vi "NEW_PRN Generation_Station1.vi"(8 "error in (no error)":errorcluster, 11 "ClusterIN":T2) -> (0 "error out":errorcluster, 2 "ClusterOUT":T2)   [LabVIEW 2017]
uses:
  <vilib>/addons/database/Connection.llb/Conn ObjectReference.ctl
  <vilib>/addons/database/NI_Database_API.lvlib
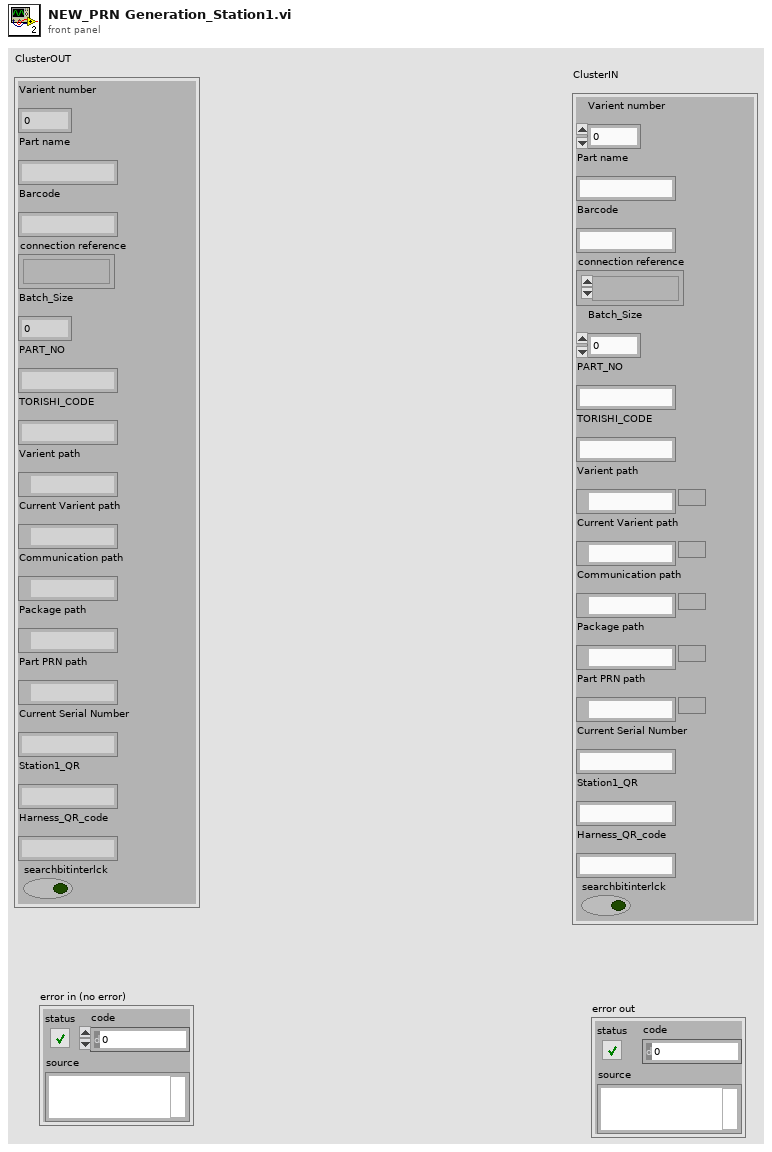
[diagram p1: front panel]
types:
  T1 = typedef "NI_Database_API.lvlib/Conn ObjectReference.ctl" = refnum<k1>
  T2 = cluster{"Varient number":u16, "Part name":string, "Barcode":string, "connection reference":T1, "Batch_Size":u16, "PART_NO":string, "TORISHI_CODE":string, "Varient path":path, "Current Varient path":path, "Communication path":path, "Package path":path, "Part PRN path":path, "Current Serial Number":string, "Station1_QR":string, "Harness_QR_code":string, "searchbitinterlck":bool}
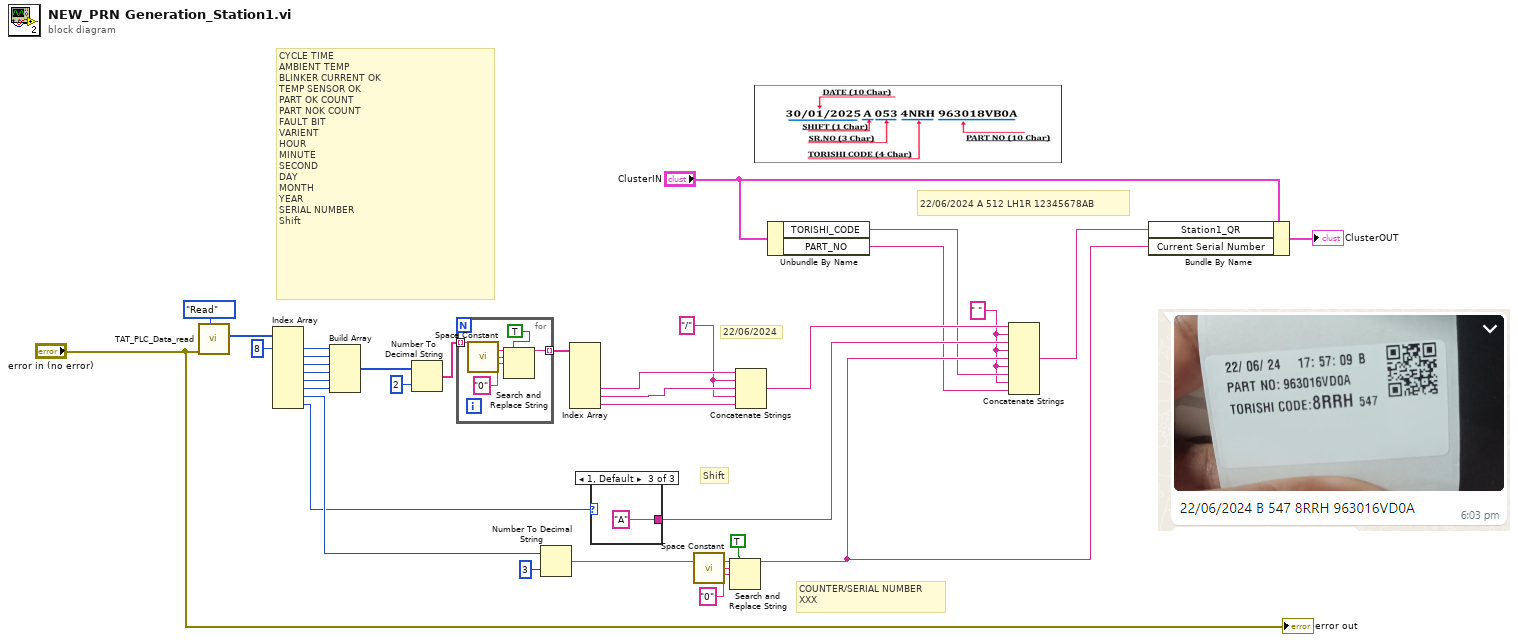
[diagram p0: block diagram]
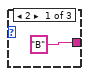
[diagram p2: hidden frame]
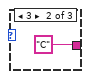
[diagram p3: hidden frame]
diagram:
  w4 = " " ("string")
  w9 = "/" ("string")
  # "22/06/2024 A 512 LH1R 12345678AB"
  # "22/06/2024"
  # "CYCLE TIME\nAMBIENT TEMP\nBLINKER CURRENT OK\nTEMP SENSOR OK\nPART OK COUNT\nPART NOK COUNT\nFAULT BIT\nVARIENT\nHOUR\nMINUTE\nSECOND\nDAY\nMONTH\nYEAR\nSERIAL NUMBER\nShift"
  # "COUNTER/SERIAL NUMBER\nXXX"
  # "Shift"
  n1 = call "TAT_PLC_Data_read.vi"("Enum"=enum16{"Read", "Write"}."Read", "error in (no error)"="error in (no error)") -> ("Array 2"=w24:u16[])  [unwired: 8 in, 1 out]
  n2 = Index Array(array=w24, index #1=8 ("index")) -> (element #1=w21:u16, element #2=w20:u16, element #3=w19:u16, element #4=w18:u16, element #5=w17:u16, element #6=w16:u16, element #7=w14:u16, element #8=w2:u16)  [unwired: 7 in]
  n3 = Build Array(w21, w20, w19, w18, w17, w16) -> (w15:u16[])
  n4 = Number To Decimal String(number=w15, width (-)=i16 2) -> (decimal integer string=w29:string[])
  n5 = for {
    tunnel: w29 -> [w36] mode=indexing
    tunnel: [w35] -> w28 mode=indexing
    n6 = call <vilib>:"Space Constant.vi"() -> ("String"=w37:string)
    n7 = Search and Replace String(replace all?=TRUE ("replace all? (F)"), input string=w36, search string=w37, replace string="0" ("replace string (\"\")")) -> (result string=w35:string)  [unwired: 4 in, 3 out]
  }
  n8 = Number To Decimal String(number=w14, width (-)=i16 3) -> (decimal integer string=w12:string)
  n9 = Index Array(array=w28) -> (element #4=w11:string, element #5=w13:string, element #6=w10:string)  [unwired: 6 in, 3 out]
  n10 = case shown="1, Default" w2 {
    tunnel: ["B" "C" "A"] -> w7
    frame 2 {
    }
    frame 3 {
    }
    frame 1, Default {
    }
  }
  n11 = call <vilib>:"Space Constant.vi"() -> ("String"=w31:string)
  n12 = Search and Replace String(replace all?=TRUE ("replace all? (F)"), input string=w12, search string=w31, replace string="0" ("replace string (\"\")")) -> (result string=w6:string)  [unwired: 4 in, 3 out]
  n13 = Concatenate Strings(w11, w9, w13, w9, w10) -> (w8:string)
  n14 = Unbundle By Name("ClusterIN") -> ("TORISHI_CODE"=w5:string, "PART_NO"=w1:string)
  n15 = Concatenate Strings(w8, w4, w7, w4, w6, w4, w5, w4, w1) -> (w3:string)
  n16 = Bundle By Name(cluster="ClusterIN", "Station1_QR"=w3, "Current Serial Number"=w6) -> (→"ClusterOUT":T2)
  "error out" <- "error in (no error)"
